vi "Build VI Description Command.vi"(8 "error in (no error)":errorcluster, 11 "Test in":refnum<class "Test.lvclass">) -> (0 "error out":errorcluster, 2 "VI Description Command":string)   [LabVIEW 2018, in "Test.lvclass"]
doc: "Builds the state machine command to configure and add the VI Description to the newly created assert vi"
uses:
  Test.lvclass
  Test Class String IDs.vi
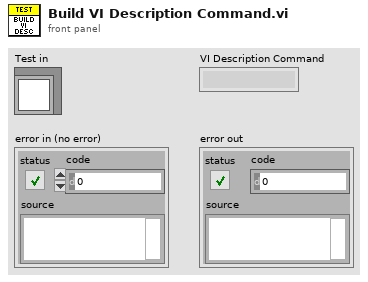
[diagram p1: front panel]
types:
  T1 = cluster{"Comparison Value 1":string, "Comparison Value 2":string, "Invert Result":string, "Assert VI Name":string, "Data Type":string, "Builder User Name":string, "Build Timestamp":string, "Failure Action":string, "Comment":string, "Assert Name":string, "Description":string, "Evaluation String":string}
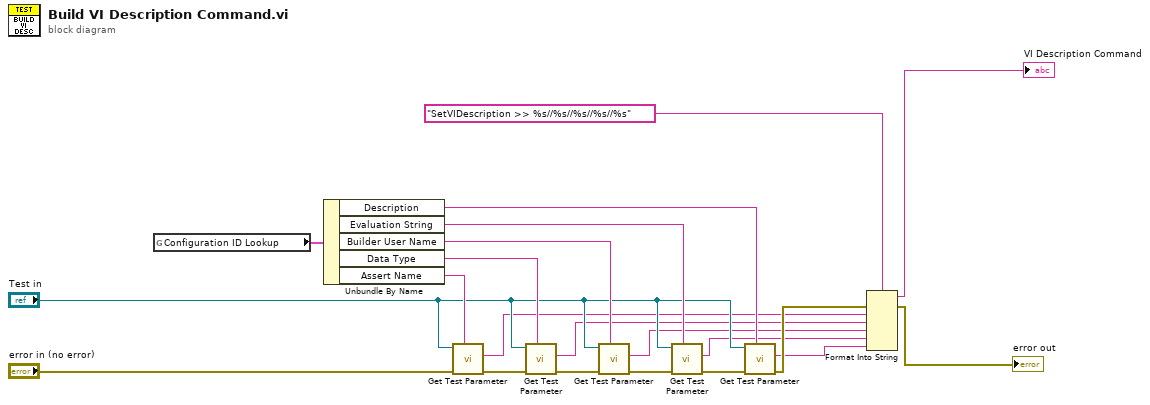
[diagram p0: block diagram]
diagram:
  n1 = global read "Test Class String IDs.vi" "Configuration ID Lookup"() -> (w14:T1)
  n2 = Unbundle By Name(w14) -> ("Description"=w19:string, "Evaluation String"=w18:string, "Builder User Name"=w17:string, "Data Type"=w16:string, "Assert Name"=w15:string)
  n3 = call "Get Test Parameter.vi"("Data Value ID"=w15, "error in (no error)"="error in (no error)", "Test in"="Test in") -> ("error out"=w3:errorcluster, "Test Parameter"=w11:string)  [unwired: 6 in, 1 out]
  n4 = call "Get Test Parameter.vi"("Data Value ID"=w16, "error in (no error)"=w3, "Test in"="Test in") -> ("error out"=w5:errorcluster, "Test Parameter"=w12:string)  [unwired: 6 in, 1 out]
  n5 = call "Get Test Parameter.vi"("Data Value ID"=w17, "error in (no error)"=w5, "Test in"="Test in") -> ("error out"=w2:errorcluster, "Test Parameter"=w7:string)  [unwired: 6 in, 1 out]
  n6 = call "Get Test Parameter.vi"("Data Value ID"=w18, "error in (no error)"=w2, "Test in"="Test in") -> ("error out"=w4:errorcluster, "Test Parameter"=w8:string)  [unwired: 6 in, 1 out]
  n7 = call "Get Test Parameter.vi"("Data Value ID"=w19, "error in (no error)"=w4, "Test in"="Test in") -> ("error out"=w20:errorcluster, "Test Parameter"=w9:string)  [unwired: 6 in, 1 out]
  n8 = Format Into String(format string="SetVIDescription >> %s//%s//%s//%s//%s" ("Append Element(s)"), error in=w20, w11, w12, w7, w8, w9) -> (resulting string=→"VI Description Command":string, error out=→"error out":errorcluster)  [unwired: 1 in]
